vi "save AutoCad cmds.vi"(5 "File name suffix":string, 7 "DesignRequest":T1, 10 "error in":errorcluster, 11 "AC.txt":string) -> (2 "error out":errorcluster)   [LabVIEW 2012, in "Design Server.lvlib"]
uses:
  Design Server.lvlib
  Design Request.ctl
  Variable cluster.ctl
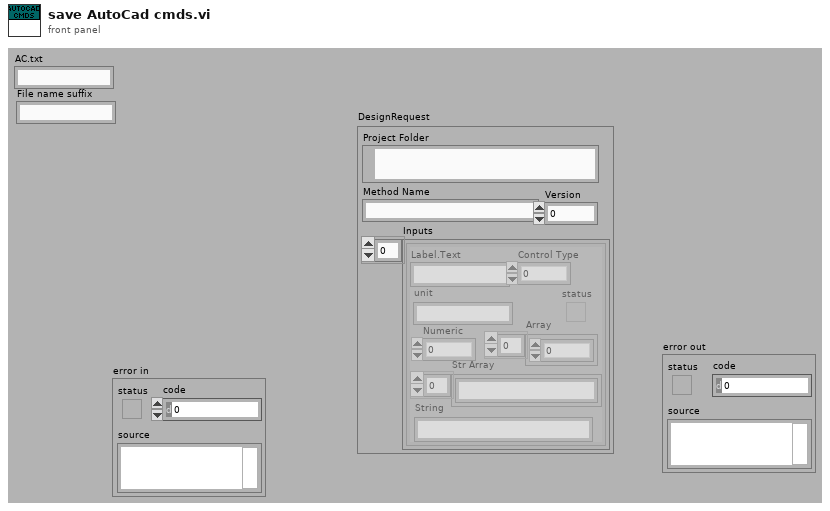
[diagram p1: front panel]
types:
  T1 = typedef "Design Server.lvlib/Design Request.ctl" = cluster{"Project Folder":path, "Method Name":string, "Inputs":T2, "Version":i32}
  T2 = typedef "Design Server.lvlib/Variable cluster.ctl" = cluster{"Label.Text":string, "Control Type":u32, "Numeric":dbl, "Array":dbl[], "status":bool, "Str Array":string[], "String":string, "unit":string}[]
  T3 = enum16{"open", "replace", "create", "open or create", "replace or create", "replace or create with confirmation"}
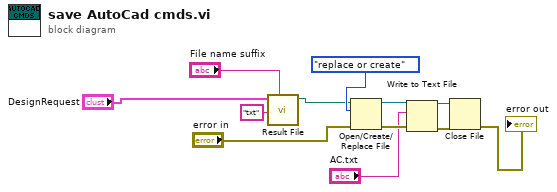
[diagram p0: block diagram]
diagram:
  n1 = call "Result File.vi"("File name suffix"="File name suffix", "File Type"="txt", "DesignRequest"="DesignRequest") -> ("File path"=w6:path)  [unwired: 7 in, 1 out]
  n2 = Open/Create/Replace File(file path (use dialog)=w6, error in="error in", operation (0:open)=T3."replace or create") -> (refnum out=w9:refnum<file>, error out=w8:errorcluster)  [unwired: 3 in, 1 out]
  n3 = Write to Text File(file (use dialog)=w9, text="AC.txt", error in=w8) -> (refnum out=w10:refnum<file>, error out=w11:errorcluster)  [unwired: 1 in, 1 out]
  n4 = Close File(refnum=w10, error in=w11) -> (error out=→"error out":errorcluster)  [unwired: 1 out]
